vi "UHR-Fleezers Control (host) -Leonardo 04-2018 V2.vi"(0 "Tab Control":T5(tab)=enum."Trap Control (RF)") -> ()   [LabVIEW 2013] (continued)
        n486 = xnode "Read/Write Control"("FPGA VI Reference In"=w836, "error in"=w835, "+ phase"=w832) -> ("error out"=w831:errorcluster)  [unwired: 1 out]
      }
      event "Signals to Plot": Double Click {
        w844 = u32 9868950 ("Color Box")
        n487 = event-data() -> ("Row"=w846:i32)  [unwired: 9 out]
        n488 = property on="All Signals" class="WFChart (strict)"("Active Plot"=w846) -> (error out=w857:errorcluster)  [unwired: 2 in, 1 out]
        n489 = property on="All Signals" class="WFChart (strict)" props=["Plot", "Visible?", "Plot", "Plot Color"](error in=w857) -> (error out=w856:errorcluster, "Plot.Visible?"=w855:bool)  [unwired: 1 in, 2 out]
        n490 = Select(t=FALSE ("Plot.Visible"), s=w855, f=TRUE ("Plot.Visible")) -> (s? t:f=w850:bool)
        n491 = property on="All Signals" class="WFChart (strict)"(error in=w856, "Plot.Visible?"=w850) -> (error out=w852:errorcluster)  [unwired: 1 in, 1 out]
        n492 = property on="All Signals" class="WFChart (strict)"(error in=w852) -> (error out=w847:errorcluster, "Plot.Plot Color"=w851:u32)  [unwired: 1 in, 1 out]
        n493 = property on="Signals to Plot" class="LstBox (strict)"(error in=w847, "Active Row"=w846) -> (error out=w845:errorcluster)  [unwired: 1 in, 1 out]
        n494 = Select(t=w851, s=w850, f=u32 0) -> (s? t:f=w848:u32)
        n495 = property on="Signals to Plot" class="LstBox (strict)"(error in=w845, "CellFontColor"=w848, "SelColor"=w844, "CellBG"=w844, "CellFontSize"=u32 20 ("Active Row:Cell Font:Size"), "CellFontBold"=TRUE ("Active Row:Cell Font:Bold")) -> ()  [unwired: 1 in, 2 out]
      }
      event "Dynamic Force FB": Value Change {
        n496 = event-data() -> ()  [unwired: 7 out]
        n497 = xnode "Read/Write Control"("FPGA VI Reference In"=w859, "Dynamic Force FB (Ronen)"="Dynamic Force FB") -> ()  [unwired: 1 in, 2 out]
      }
      event "BD 1 Frequency 1 (MHz)", "BD 1 Frequency 2 (MHz)", "BD 1 Frequency 3 (MHz)", "BD 2 Frequency 1 (MHz)", "BD 2 Frequency 2 (MHz)", "BD 2 Frequency 3 (MHz)", "Trap Delta (MHz)": Value Change {
        # "anytime one of the frequencies is changed, write it to the RF board UNLESS Set 2 is being oscillated. The oscillation\nscript writes the frequencies to the RF board."
        n498 = event-data() -> ("CtlRef"=w862:refnum<vi>)  [unwired: 6 out]
        n499 = control-ref of="Trap Delta (MHz)"() -> (w861:refnum<vi>)
        n500 = Equal?(x=w861, y=w862) -> (x = y?=w860:bool)
        n501 = case shown="False" "Oscillate Set 2" {
          tunnel: w865 -> [w886 _]
          tunnel: [w885 w898] -> w864
          tunnel: w863 -> [w884 w898]
          tunnel: w860 -> [w871 _]
          frame False {
            n502 = case shown="False" "Symmetric manual \ntrap motion" {
              tunnel: ["T2 for asymmetric\n(MHz)" w897] -> w872
              tunnel: "Trap Delta (MHz)" -> [w891 w896]
              tunnel: [w890 w893] -> w868
              frame False {
                n503 = Subtract(x="T2 for asymmetric\n(MHz)", y=w891) -> (x-y=w890:dbl)
              }
              frame True {
                n504 = Divide(x=w896, y=2) -> (x/y=w894:dbl)
                n505 = Subtract(x="Middle freq for \nsymmetric (MHz)", y=w894) -> (x-y=w893:dbl)
                n506 = Add(x="Middle freq for \nsymmetric (MHz)", y=w894) -> (x+y=w897:dbl)
              }
            }
            n507 = local read "BD 1 Frequency 2 (MHz)"() -> (w873:dbl)
            n508 = local write "BD 1 Frequency 1 (MHz)"(w868) -> ()
            n509 = Select(t=w872, s=w871, f=w873) -> (s? t:f=w870:dbl)
            n510 = local read "Y RF Frequency Limits (MHz)"() -> (w874:T16)
            n511 = local read "X RF Frequency Limits (MHz)"() -> (w875:T16)
            n512 = local read "BD 1 Frequency 3 (MHz)"() -> (w887:dbl)
            n513 = local write "BD 1 Frequency 2 (MHz)"(w870) -> ()
            n514 = local read "BD 2 Frequency 1 (MHz)"() -> (w878:dbl)
            n515 = local read "BD 2 Frequency 2 (MHz)"() -> (w877:dbl)
            n516 = local read "BD 2 Frequency 3 (MHz)"() -> (w888:dbl)
            n517 = call "set RF board frequency - interlace.vi"("Board 2 Frequency Limits"=w874, "Board 1 Frequency Limits"=w875, "error in"=w884, "FPGA VI Reference In"=w886, "Board 2 Frequency 3 (MHz)"=w888, "Board 1 Frequency 3 (MHz)"=w887, "Board 2 Frequency 2 (MHz)"=w877, "Board 2 Frequency 1 (MHz)"=w878, "Board 1 Frequency 2 (MHz)"=w870, "Board 1 Frequency 1  (MHz)"=w868) -> ("error out"=w885:errorcluster)  [unwired: 1 out]
            n518 = Subtract(x=w878, y=w877) -> (x-y=w882:dbl)
            n519 = Subtract(x=w870, y=w868) -> (x-y=w883:dbl)
            n520 = Square(x=w882) -> (x^2=w880:dbl)
            n521 = Square(x=w883) -> (x^2=w881:dbl)
            n522 = Add(x=w881, y=w880) -> (x+y=w879:dbl)
            n523 = Square Root(x=w879) -> (sqrt(x)=w876:dbl)
            n524 = local write "Trap Delta (MHz)"(w876) -> ()
            n525 = property on="Initial delta (MHz)" class="DigNum (strict)"("Val(Sgnl)"=w876) -> ()  [unwired: 2 in, 2 out]
          }
          frame True {
          }
        }
      }
      event "Round T1 X": Value Change {
        n526 = event-data() -> ()  [unwired: 7 out]
        n527 = local read "BD 1 Frequency 1 (MHz)"() -> (w901:dbl)
        n528 = Round To Nearest(number=w901) -> (nearest integer value=w900:dbl)
        n529 = property on="BD 1 Frequency 1 (MHz)" class="DigNum (strict)"("Val(Sgnl)"=w900) -> ()  [unwired: 2 in, 2 out]
      }
      event "Round T2 X": Value Change {
        n530 = event-data() -> ()  [unwired: 7 out]
        n531 = local read "BD 1 Frequency 2 (MHz)"() -> (w903:dbl)
        n532 = Round To Nearest(number=w903) -> (nearest integer value=w902:dbl)
        n533 = property on="BD 1 Frequency 2 (MHz)" class="DigNum (strict)"("Val(Sgnl)"=w902) -> ()  [unwired: 2 in, 2 out]
      }
      event "Stop All": Value Change {
        n534 = event-data() -> ()  [unwired: 7 out]
        n535 = call "hamilton_controller.vi"("action"=T21."DISCONNECT") -> ()  [unwired: 10 in, 1 out]
        n536 = local read "Stop All"() -> (w906:bool)
      }
      event "Delayed Interlace Start": Value Change {
        n537 = event-data() -> ()  [unwired: 7 out]
        n538 = flat-sequence {
          frame #0 {
            n539 = Multiply(x="Delay to Interlace (s)", y=1000.0) -> (x*y=w909:dbl)
            n540 = Wait (ms)(milliseconds to wait=w909) -> ()  [unwired: 1 out]
          }
          frame #1 {
            n541 = property on="Green laser mode" class="RadioBtnsControl (strict)"("Val(Sgnl)"=enum32{"Laser ON", "Laser OFF", "Interlace"}."Interlace" ("Value (Signaling)")) -> ()  [unwired: 2 in, 2 out]
          }
        }
      }
      event "BD 1 Amplitude 1 (%)", "BD 1 Amplitude 2 (%)", "BD 1 Amplitude 3 (%)", "BD 2 Amplitude 1 (%)", "BD 2 Amplitude 2 (%)", "BD 2 Amplitude 3 (%)", "Trap 1 ON", "Trap 2 ON", "Trap 3 ON", "Feedback On/Off", "All FB On/Off": Value Change {
        w933 = i16 1 ("f")
        n542 = event-data() -> ()  [unwired: 7 out]
        n543 = local write "Trap 1 (ON/OFF)"("Trap 1 ON") -> ()
        n544 = local write "Trap 2 (ON/OFF)"("Trap 2 ON") -> ()
        n545 = Boolean To (0,1)(Boolean="Trap 3 ON") -> (0, 1=w934:i16)
        n546 = Boolean To (0,1)(Boolean="Trap 1 ON") -> (0, 1=w935:i16)
        n547 = Boolean To (0,1)(Boolean="Trap 2 ON") -> (0, 1=w936:i16)
        n548 = Select(t=w936, s="Trap ON/OFF X or Y Amp?", f=w933) -> (s? t:f=w931:i16)
        n549 = Select(t=w935, s="Trap ON/OFF X or Y Amp?", f=w933) -> (s? t:f=w932:i16)
        n550 = Select(t=w934, s="Trap ON/OFF X or Y Amp?", f=w933) -> (s? t:f=w930:i16)
        n551 = Select(t=w933, s="Trap ON/OFF X or Y Amp?", f=w936) -> (s? t:f=w928:i16)
        n552 = Select(t=w933, s="Trap ON/OFF X or Y Amp?", f=w935) -> (s? t:f=w929:i16)
        n553 = Select(t=w933, s="Trap ON/OFF X or Y Amp?", f=w934) -> (s? t:f=w927:i16)
        n554 = And(x="All FB On/Off", y="Feedback On/Off") -> (x .and. y?=w925:cluster{"Set 1":bool, "Set 2":bool})
        n555 = local read "BD 1 Amplitude 1 (%)"() -> (w945:dbl)
        n556 = local read "BD 1 Amplitude 2 (%)"() -> (w944:dbl)
        n557 = local read "BD 1 Amplitude 3 (%)"() -> (w943:dbl)
        n558 = Unbundle By Name(w925) -> ("Set 1"=w921:bool, "Set 2"=w918:bool)
        n559 = local read "Y RF Amplitude Limits (%)"() -> (w914:T16)
        n560 = local read "X RF Amplitude Limits (%)"() -> (w915:T16)
        n561 = local read "BD 2 Amplitude 1 (%)"() -> (w946:dbl)
        n562 = local read "BD 2 Amplitude 2 (%)"() -> (w947:dbl)
        n563 = local read "BD 2 Amplitude 3 (%)"() -> (w948:dbl)
        n564 = And(x="Trap 2 ON", y=w918) -> (x .and. y?=w916:bool)
        n565 = And(x="Trap 1 ON", y=w921) -> (x .and. y?=w919:bool)
        n566 = Multiply(x=w932, y=w945) -> (x*y=w940:dbl)
        n567 = Multiply(x=w944, y=w931) -> (x*y=w938:dbl)
        n568 = Multiply(x=w943, y=w930) -> (x*y=w939:dbl)
        n569 = Multiply(x=w946, y=w929) -> (x*y=w949:dbl)
        n570 = Multiply(x=w947, y=w928) -> (x*y=w950:dbl)
        n571 = Multiply(x=w948, y=w927) -> (x*y=w951:dbl)
        n572 = call "set RF board amplitude - interlace.vi"("Board 2 Amplitude Limits"=w914, "Board 1 Amplitude Limits"=w915, "error in"=w941, "FPGA VI Reference In"=w942, "Board 2 Amplitude 3 (%)"=w951, "Board 1 Amplitude 3 (%)"=w939, "Board 2 Amplitude 2 (%)"=w950, "Board 2 Amplitude 1 (%)"=w949, "Board 1 Amplitude 2 (%)"=w938, "Board 1 Amplitude 1 (%)"=w940) -> ("error out"=w923:errorcluster, "FPGA VI Reference Out"=w924:T20)
        n573 = xnode "Read/Write Control"("FPGA VI Reference In"=w924, "error in"=w923, "FB On/Off Set 1"=w919, "FB On/Off Set 2"=w916) -> ("error out"=w922:errorcluster)  [unwired: 1 out]
        n574 = case shown="True" "All FB On/Off" {
          frame False {
          }
          frame True {
            n575 = local write "Feedback overload"(FALSE) -> ()
          }
        }
      }
      event "Load parameters": Value Change {
        n576 = event-data() -> ()  [unwired: 7 out]
        n577 = property on="Saved AOD Raster Scan Parameter Sets" class="Arr (strict)"() -> ("Index Values"=w963:u32[])  [unwired: 2 in, 2 out]
        n578 = Index Array(array=w963, index=0) -> (element=w960:u32)
        n579 = local write "Load parameters"(FALSE ("Load parameters")) -> ()
        n580 = Index Array(array="Saved AOD Raster Scan Parameter Sets", index=w960) -> (element=w959:T31)
        n581 = Unbundle By Name(w959) -> ("Scan Range AOD (nm) 2"=w958:dbl, "Step Size AOD (nm) 2"=w957:dbl, "Scan Speed AOD (nm/s) 2"=w956:dbl, "Number of scans (AOD) 2"=w955:u16)
        n582 = flat-sequence {
          tunnel: w958 -> [w966]
          tunnel: w957 -> [w965]
          tunnel: w956 -> [w964]
          tunnel: w955 -> [w967]
          frame #0 {
            n583 = local write "Scan Speed (nm/s)"(w964) -> ()
            n584 = local write "Scan Range (nm)"(w966) -> ()
            n585 = local write "Step Size (nm)"(w965) -> ()
          }
          frame #1 {
            n586 = property on="Number of F/B Scans (AOD)" class="DigNum (strict)"("Val(Sgnl)"=w967) -> ()  [unwired: 2 in, 2 out]
          }
        }
      }
      event "Trap 1 (ON/OFF)", "Trap 2 (ON/OFF)": Value Change {
        n587 = event-data() -> ()  [unwired: 7 out]
        n588 = property on="Trap 2 ON" class="Bool (strict)"("Val(Sgnl)"="Trap 2 (ON/OFF)") -> ()  [unwired: 2 in, 2 out]
        n589 = property on="Trap 1 ON" class="Bool (strict)"("Val(Sgnl)"="Trap 1 (ON/OFF)") -> ()  [unwired: 2 in, 2 out]
      }
      event "DIO count 1 (ticks)", "DIO count 2 (ticks)", "DIO count 3 (ticks)", "Interlace", "Number Interlace Sets", "Not-Interlacing Set": Value Change {
        n590 = event-data() -> ()  [unwired: 7 out]
        n591 = local read "DIO count 3 (ticks)"() -> (w980:u32)
        n592 = local read "DIO count 1 (ticks)"() -> (w982:u32)
        n593 = local read "DIO count 2 (ticks)"() -> (w981:u32)
        n594 = To Unsigned Byte Integer(number="Not-Interlacing Set") -> (unsigned 8bit integer=w971:u8)
        n595 = Add(x=w971, y=u8 1) -> (x+y=w975:u8)
        n596 = xnode "Read/Write Control"("FPGA VI Reference In"=w986, "error in"=w984, "DIO count 1 (ticks)"=w982, "DIO count 2 (ticks)"=w981, "DIO count 3 (ticks)"=w980, "Interlace ON/OFF"="Interlace", "Number Interlace Cycles"="Number Interlace Sets", "Interlace Off Parameters"=w975) -> ("error out"=w985:errorcluster)  [unwired: 1 out]
        n597 = Build Array(w982, w981, w980) -> (w973:u32[])
        n598 = Split 1D Array(array=w973, index="Number Interlace Sets") -> (first subarray=w983:u32[])  [unwired: 1 out]
        n599 = Index Array(array=w973, index=w971) -> (element=w972:u32)
        n600 = Add Array Elements(numeric array=w983) -> (sum=w977:u32)
        n601 = Select(t=w977, s="Interlace", f=w972) -> (s? t:f=→"Total Counts (ticks)":u32)
      }
      event "Reset Feedback": Value Change {
        n602 = event-data() -> ()  [unwired: 7 out]
        n603 = Unbundle By Name("Reset Feedback") -> ("Set 1"=w990:bool, "Set 2"=w989:bool)
        n604 = xnode "Read/Write Control"("FPGA VI Reference In"=w992, "error in"=w987, "FB Reset Set 1"=w990, "FB Reset Set 2"=w989) -> ("error out"=w988:errorcluster)  [unwired: 1 out]
      }
      event "PID gains": Value Change {
        n605 = event-data() -> ()  [unwired: 7 out]
        n606 = local read "PID gains"() -> (w993:T10)
        n607 = xnode "Read/Write Control"("FPGA VI Reference In"=w996, "error in"=w994, "FB Gains"=w993) -> ("error out"=w995:errorcluster)  [unwired: 1 out]
      }
      event "AI2 to Setpoint", "Trap Intensity\nSetpoints (V)": Value Change {
        n608 = event-data() -> ()  [unwired: 7 out]
        n609 = xnode "Read/Write Control"("FPGA VI Reference In"=w1001, "error in"=w997) -> ("FPGA VI Reference Out"=w1000:T20, "error out"=w999:errorcluster, "AI2 Y Sum Set 1"=w1008:i16, "AI2 Y Sum Set 2"=w1007:i16)
        n610 = Cluster To Array(cluster="AI2 to Setpoint") -> (array=w1011:bool[])
        n611 = local read "AI2 (V)"() -> (w1009:cluster{"Set 1":dbl, "Set 2":dbl})
        n612 = Or Array Elements(Boolean array=w1011) -> (logical OR=w1012:bool)
        n613 = Bundle By Name(cluster=w1009, "Set 1"=w1008, "Set 2"=w1007) -> (w1006:cluster{"Set 1":dbl, "Set 2":dbl})
        n614 = Divide(x=w1006, y=3276.7) -> (x/y=w1005:cluster{"Set 1":dbl, "Set 2":dbl})
        "AI2 (V)" <- w1005
        n615 = case shown="False" w1012 {
          tunnel: [w1015 w1032] -> w1004
          tunnel: "AI2 to Setpoint" -> [_ w1028]
          tunnel: "Trap Intensity\nSetpoints (V)" -> [w1016 w1031]
          tunnel: w1005 -> [_ w1025]
          frame False {
            n616 = Multiply(x=3276.7, y=w1016) -> (x*y=w1017:cluster{"Set 1":dbl, "Set 2":dbl})
            n617 = To Word Integer(number=w1017) -> (16bit integer=w1015:cluster{"Set 1":i16, "Set 2":i16})
          }
          frame True {
            n618 = Unbundle By Name(w1025) -> ("Set 1"=w1024:dbl, "Set 2"=w1023:dbl)
            n619 = Unbundle By Name(w1031) -> ("Set 1"=w1030:dbl, "Set 2"=w1029:dbl)
            n620 = Unbundle By Name(w1028) -> ("Set 1"=w1027:bool, "Set 2"=w1026:bool)
            n621 = Select(t=w1024, s=w1027, f=w1030) -> (s? t:f=w1022:dbl)
            n622 = Select(t=w1023, s=w1026, f=w1029) -> (s? t:f=w1021:dbl)
            n623 = Bundle By Name(cluster=w1031, "Set 1"=w1022, "Set 2"=w1021) -> (w1019:cluster{"Set 1":dbl, "Set 2":dbl})
            n624 = local write "Trap Intensity\nSetpoints (V)"(w1019) -> ()
            n625 = Multiply(x=3276.7, y=w1019) -> (x*y=w1020:cluster{"Set 1":dbl, "Set 2":dbl})
            n626 = To Word Integer(number=w1020) -> (16bit integer=w1032:cluster{"Set 1":i16, "Set 2":i16})
          }
        }
        n627 = Unbundle By Name(w1004) -> ("Set 1"=w1003:i16, "Set 2"=w1002:i16)
        n628 = xnode "Read/Write Control"("FPGA VI Reference In"=w1000, "error in"=w999, "FB Setpoint Set 1"=w1003, "FB Setpoint Set 2"=w1002) -> ("error out"=w998:errorcluster)  [unwired: 1 out]
      }
      event "Invert GI": Value Change {
        n629 = event-data() -> ()  [unwired: 7 out]
        n630 = xnode "Read/Write Control"("FPGA VI Reference In"=w1037, "error in"=w1035, "Invert GI"="Invert GI", "Invert GI 2"="Invert GI") -> ("error out"=w1036:errorcluster)  [unwired: 1 out]
      }
      event "Green FB Setpoint (mV)", "Green FB Gains", "Green FB On/Off", "Current When FB OFF (%)", "Green int current ON count adj": Value Change {
        n631 = event-data() -> ()  [unwired: 7 out]
        n632 = local read "Green FB Setpoint (mV)"() -> (w1044:dbl)
        n633 = local read "Current When FB OFF (%)"() -> (w1047:dbl)
        n634 = Multiply(x=w1044, y=3.2767) -> (x*y=w1043:dbl)
        n635 = Multiply(x=w1047, y=655.35) -> (x*y=w1048:dbl)
        n636 = To Unsigned Word Integer(number=w1048) -> (unsigned 16bit integer=w1046:u16)
        n637 = local read "Green int current ON count adj"() -> (w1051:u32)
        n638 = local read "Green FB Gains"() -> (w1050:T10)
        n639 = local read "Green Laser ON/Interlacing"() -> (w1041:bool)
        n640 = local read "Green laser mode"() -> (w1040:enum32{"Laser ON", "Laser OFF", "Interlace"})
        n641 = local read "Green FB On/Off"() -> (w1052:bool)
        n642 = Equal?(x=w1040, y=enum32{"Laser ON", "Laser OFF", "Interlace"}."Interlace") -> (x = y?=w1038:bool)
        n643 = Compound Arithmetic op=AND(w1038, w1052, w1041) -> (w1042:bool)
        n644 = xnode "Read/Write Control"("FPGA VI Reference In"=w1055, "error in"=w1054, "Green FB Setpoint"=w1043, "Green FB On/Off"=w1042, "Current Out"=w1046, "Green int current ON count adj"=w1051, "Green FB Gains"=w1050) -> ("error out"=w1053:errorcluster)  [unwired: 1 out]
      }
      event "Green laser mode", "Green Laser ON/Interlacing": Value Change {
        n645 = event-data() -> ()  [unwired: 7 out]
        n646 = case shown="True" "Green Laser ON/Interlacing" {
          tunnel: "Green laser mode" -> [_ w1069]
          tunnel: [enum32{"Laser ON", "Laser OFF", "Interlace"}."Laser OFF" ("Green laser mode") w1069] -> w1057
          tunnel: [FALSE w1065] -> w1056
          frame False {
          }
          frame True {
            n647 = local read "Green FB On/Off"() -> (w1066:bool)
            n648 = Equal?(x=w1069, y=enum32{"Laser ON", "Laser OFF", "Interlace"}."Interlace") -> (x = y?=w1067:bool)
            n649 = And(x=w1067, y=w1066) -> (x .and. y?=w1065:bool)
          }
        }
        n650 = xnode "Read/Write Control"("FPGA VI Reference In"=w1062, "error in"=w1060, "Operating Mode"=w1057, "Operating Mode 2"=w1057, "Green FB On/Off"=w1056) -> ("error out"=w1061:errorcluster)  [unwired: 1 out]
      }
      event "- phase (APD 1 Gate)", "+ phase (APD 1 Gate)": Value Change {
        n651 = event-data() -> ()  [unwired: 7 out]
        n652 = local read "Phase Adj. (APD 1 Gate)"() -> (w1070:i16)
        n653 = Negate(x=w1070) -> (-x=w1078:i16)
        n654 = Select(t=w1078, s="- phase (APD 1 Gate)", f=w1070) -> (s? t:f=w1077:i16)
        n655 = Or(x="- phase (APD 1 Gate)", y="+ phase (APD 1 Gate)") -> (x .or. y?=w1073:bool)
        n656 = xnode "Read/Write Control"("FPGA VI Reference In"=w1080, "error in"=w1079, "Phase count adjustment (APD 1 Gate)"=w1077) -> ("FPGA VI Reference Out"=w1075:T20, "error out"=w1076:errorcluster)
        n657 = xnode "Read/Write Control"("FPGA VI Reference In"=w1075, "error in"=w1076, "+ phase (APD 1 Gate)"=w1073) -> ("error out"=w1074:errorcluster)  [unwired: 1 out]
      }
      event "Phase Adj. (APD Acq)", "+ phase (APD Acq)", "- phase (APD Acq)": Value Change {
        n658 = event-data() -> ()  [unwired: 7 out]
        n659 = local read "Phase Adj. (APD Acq)"() -> (w1083:i16)
        n660 = Negate(x=w1083) -> (-x=w1089:i16)
        n661 = Select(t=w1089, s="+ phase (APD Acq)", f=w1083) -> (s? t:f=w1088:i16)
        n662 = Or(x="+ phase (APD Acq)", y="- phase (APD Acq)") -> (x .or. y?=w1084:bool)
        n663 = xnode "Read/Write Control"("FPGA VI Reference In"=w1091, "error in"=w1090, "Phase Count Adjustment (APD Acq)"=w1088) -> ("FPGA VI Reference Out"=w1086:T20, "error out"=w1087:errorcluster)
        n664 = xnode "Read/Write Control"("FPGA VI Reference In"=w1086, "error in"=w1087, "+ phase (APD Acq)"=w1084) -> ("error out"=w1085:errorcluster)  [unwired: 1 out]
      }
      event "Phase adj. (GI)", "+ phase (GI)", "- phase (GI)": Value Change {
        n665 = event-data() -> ()  [unwired: 7 out]
        n666 = Negate(x="Phase adj. (GI)") -> (-x=w1100:i16)
        n667 = Select(t=w1100, s="+ phase (GI)", f="Phase adj. (GI)") -> (s? t:f=w1099:i16)
        n668 = Or(x="+ phase (GI)", y="- phase (GI)") -> (x .or. y?=w1095:bool)
        n669 = xnode "Read/Write Control"("FPGA VI Reference In"=w1102, "error in"=w1101, "Phase count adjustment (GI)"=w1099) -> ("FPGA VI Reference Out"=w1097:T20, "error out"=w1098:errorcluster)
        n670 = xnode "Read/Write Control"("FPGA VI Reference In"=w1097, "error in"=w1098, "+ phase (GI)"=w1095) -> ("error out"=w1096:errorcluster)  [unwired: 1 out]
      }
      event "Phase adj. (GI) 2", "+ phase (GI) 2", "- phase (GI) 2": Value Change {
        n671 = event-data() -> ()  [unwired: 7 out]
        n672 = Negate(x="Phase adj. (GI) 2") -> (-x=w1111:i16)
        n673 = Select(t=w1111, s="+ phase (GI) 2", f="Phase adj. (GI) 2") -> (s? t:f=w1110:i16)
        n674 = Or(x="+ phase (GI) 2", y="- phase (GI) 2") -> (x .or. y?=w1106:bool)
        n675 = xnode "Read/Write Control"("FPGA VI Reference In"=w1113, "error in"=w1112, "Phase count adjustment (GI) 2"=w1110) -> ("FPGA VI Reference Out"=w1108:T20, "error out"=w1109:errorcluster)
        n676 = xnode "Read/Write Control"("FPGA VI Reference In"=w1108, "error in"=w1109, "+ phase (GI) 2"=w1106) -> ("error out"=w1107:errorcluster)  [unwired: 1 out]
      }
      event "Phase adj. (Green FB)", "- phase (Green FB)", "+ phase (Green FB)": Value Change {
        n677 = event-data() -> ()  [unwired: 7 out]
        n678 = Negate(x="Phase adj. (Green FB)") -> (-x=w1122:i16)
        n679 = Select(t=w1122, s="+ phase (Green FB)", f="Phase adj. (Green FB)") -> (s? t:f=w1121:i16)
        n680 = Or(x="+ phase (Green FB)", y="- phase (Green FB)") -> (x .or. y?=w1117:bool)
        n681 = xnode "Read/Write Control"("FPGA VI Reference In"=w1124, "error in"=w1123, "Phase count adjustment (Green FB)"=w1121) -> ("FPGA VI Reference Out"=w1119:T20, "error out"=w1120:errorcluster)
        n682 = xnode "Read/Write Control"("FPGA VI Reference In"=w1119, "error in"=w1120, "+ phase (Green FB)"=w1117) -> ("error out"=w1118:errorcluster)  [unwired: 1 out]
      }
      event "Invert APD Gate", "APD Gate ON Count", "APD Gate OFF Count", "APD Gate", "APD Integration Time (s)", "APD 1 AO Mult.", "APD 2 AO Mult.": Value Change {
        n683 = event-data() -> ()  [unwired: 7 out]
        n684 = local read "APD Integration Time (s)"() -> (w1125:dbl)
        n685 = local read "APD Gate ON Count"() -> (w1138:u32)
        n686 = local read "APD Gate OFF Count"() -> (w1137:u32)
        n687 = local read "Invert APD Gate"() -> (w1139:bool)
        n688 = local read "APD Gate"() -> (w1136:enum32{"ON", "OFF", "Interlace"})
        n689 = Multiply(x=w1125, y=40000000.0) -> (x*y=w1134:dbl)
        n690 = Reciprocal(x=w1125) -> (1/x=→"APD Acq Rate (Hz)":dbl)
        n691 = To Unsigned Long Integer(number=w1134) -> (unsigned 32bit integer=w1133:u32)
        n692 = local read "DMA Update Period (s)"() -> (w1126:dbl)
        n693 = Divide(x=w1126, y=w1125) -> (x/y=w1129:dbl)
        n694 = local read "APD 1 AO Mult."() -> (w1131:i16)
        n695 = local read "APD 2 AO Mult."() -> (w1130:i16)
        n696 = Multiply(x=2.0, y=w1129) -> (x*y=w1128:dbl)
        n697 = local write "APD Samples/FIFO Acq."(w1129) -> ()
        n698 = local write "APD Elements/DMA read"(w1128) -> ()
        n699 = xnode "Read/Write Control"("FPGA VI Reference In"=w1142, "error in"=w1141, "Invert APD Gate"=w1139, "APD Gate ON Count"=w1138, "APD Gate OFF Count"=w1137, "APD Acq Rate Count"=w1133, "APD Gate Operating Mode"=w1136, "APD 1 AO scale factor"=w1131, "APD 2 AO scale factor"=w1130) -> ("error out"=w1140:errorcluster)  [unwired: 1 out]
      }
      event "GI Frequency, ON count", "Green FB Count", "GI Frequency, OFF count": Value Change {
        n700 = event-data() -> ()  [unwired: 7 out]
        n701 = xnode "Read/Write Control"("FPGA VI Reference In"=w1148, "error in"=w1146, "Green interlace ON count"="GI Frequency, ON count", "Green interlace OFF count"="GI Frequency, OFF count", "Green interlace ON count 2"="GI Frequency, ON count", "Green interlace OFF count 2"="GI Frequency, OFF count", "Green FB Count"="Green FB Count") -> ("error out"=w1147:errorcluster)  [unwired: 1 out]
      }
      event "Number of F/B Scans (AOD)", "Scan Speed (nm/s)", "Scan BD", "Initial delta (MHz)", "Step Size (nm)", "Scan Range (nm)": Value Change {
        w1210 = 123.0  # AOM cal (nm/MHz)
        n702 = event-data() -> ()  [unwired: 7 out]
        n703 = local read "BD 1 Frequency 1 (MHz)"() -> (w1193:dbl)
        n704 = local read "AOM X Cal (nm/MHz)"() -> (w1185:dbl)
        n705 = local read "X RF Frequency Limits (MHz)"() -> (w1197:T16)
        n706 = local read "Y RF Frequency Limits (MHz)"() -> (w1194:T16)
        n707 = local read "BD 2 Frequency 1 (MHz)"() -> (w1199:dbl)
        n708 = Negate(x="Scan Range (nm)") -> (-x=w1163:dbl)
        n709 = Divide(x=w1163, y=w1185) -> (x/y=w1167:dbl)
        n710 = Select(t=w1197, s="Scan BD", f=w1194) -> (s? t:f=w1196:T16)
        n711 = Select(t=w1193, s="Scan BD", f=w1199) -> (s? t:f=w1198:dbl)
        n712 = Unbundle By Name(w1196) -> ("Maximum"=w1205:dbl, "Minimum"=w1204:dbl)
        n713 = Add(x=w1167, y=w1198) -> (x+y=w1202:dbl)
        n714 = Divide(x=w1163, y="Step Size (nm)") -> (x/y=w1182:dbl)
        n715 = Divide(x="Step Size (nm)", y=w1185) -> (x/y=w1191:dbl)
        n716 = Absolute Value(x=w1182) -> (abs(x)=w1166:dbl)
        n717 = Sign(1:w1163) -> (0:w1164:dbl)
        n718 = In Range and Coerce(upper limit=w1205, x=w1202, lower limit=w1204) -> (coerced(x)=w1201:dbl, In Range?=w1203:bool)
        n719 = To Unsigned Quad Integer(1:w1166) -> (0:w1181:u64)
        "Scan steps (AOD)" <- w1181
        n720 = call "IR AOM freq to word.vi"("Frequency In (MHz)"=w1191) -> ("Frequency Word Out (double)"=w1188:dbl)
        n721 = Multiply(x=w1164, y=w1188) -> (x*y=w1165:dbl)
        n722 = Subtract(x=w1202, y=w1201) -> (x-y=w1200:dbl)
        n723 = To Quad Integer(1:w1165) -> (0:w1187:i64)
        "Incr. int (AOD)" <- w1187
        n724 = Subtract(x=w1167, y=w1200) -> (x-y=w1186:dbl)
        "Scan Range (MHz)" <- w1186
        n725 = Select(t=w1167, s=w1203, f=w1186) -> (s? t:f=w1206:dbl)
        n726 = Multiply(x=w1186, y=w1185) -> (x*y=w1184:dbl)
        n727 = Decrement(x=w1181) -> (x-1=w1234:u64)
        n728 = Negate(x=w1184) -> (-x=w1180:dbl)
        n729 = local write "Scan Range (nm)"(w1180) -> ()
        n730 = Divide(x=w1206, y=w1234) -> (x/y=w1190:dbl)
        "Scan Increment (MHz)" <- w1190
        n731 = call "IR AOM freq to word.vi"("Frequency In (MHz)"=w1190) -> ("Frequency Word Out (double)"=w1189:dbl)
        n732 = Divide(x="Step Size (nm)", y="Scan Speed (nm/s)") -> (x/y=w1177:dbl)
        n733 = To Quad Integer(1:w1189) -> ()  [unwired: 1 out]
        n734 = local read "Number Interlace Sets"() -> (w1161:u8)
        n735 = local read "AI Count (ticks)"() -> (w1162:u32)
        n736 = local read "Total Counts (ticks)"() -> (w1160:u32)
        n737 = local read "# Samples/trap"() -> (w1192:u32)
        n738 = Multiply(x=w1162, y=w1161) -> (x*y=w1159:u32)
        n739 = Divide(x=w1160, y=w1159) -> (x/y=w1158:dbl)
        n740 = Select(t=w1193, s="Scan BD", f=w1199) -> (s? t:f=w1231:dbl)
        "Initial freq. (MHz)" <- w1231
        n741 = Add(x=w1206, y=w1231) -> (x+y=→"Final freq. (MHz)":dbl)
        n742 = Divide(x=w1160, y=40000000.0) -> (x/y=w1176:dbl)
        n743 = Divide(x=w1177, y=w1176) -> (x/y=w1175:dbl)
        n744 = To Unsigned Quad Integer(1:w1175) -> (0:w1150:u64)
        n745 = Quotient & Remainder(x=w1150, y=u64 2) -> (x-y*floor(x/y)=w1154:u64)  [unwired: 1 out]
        n746 = Equal?(x=w1154, y=u64 0) -> (x = y?=w1152:bool)
        n747 = Decrement(x=w1150) -> (x-1=w1151:u64)
        n748 = Select(t=w1150, s=w1152, f=w1151) -> (s? t:f=w1149:u64)
        "Cycles/step (AOD)" <- w1149
        n749 = xnode "Read/Write Control"("FPGA VI Reference In"=w1242, "error in"=w1241, "Scan steps"=w1181, "Number of scans"="Number of F/B Scans (AOD)", "Cycles per step"=w1149, "Scan freq.  increment"=w1187, "Scan BD"="Scan BD") -> ("error out"=w1240:errorcluster)  [unwired: 1 out]
        n750 = Multiply(x=w1181, y=w1149) -> (x*y=w1235:u64)
        n751 = Multiply(x=w1235, y=u64 2) -> (x*y=w1157:u64)
        n752 = Multiply(x=w1158, y=w1157) -> (x*y=w1156:dbl)
        "Data points/scan (f/b)" <- w1156
        n753 = Multiply(x=w1156, y="Number of F/B Scans (AOD)") -> (x*y=w1238:dbl)
        "Data points/scans" <- w1238
        n754 = Divide(x=w1238, y=w1192) -> (x/y=→"N sets should be saved":dbl)
        n755 = Multiply(x=w1235, y=w1176) -> (x*y=w1174:dbl)
        "Time/Scan (s) (AOD)" <- w1174
        n756 = Select(t=w1206, s="Scan BD", f=0.0) -> (s? t:f=w1232:dbl)
        n757 = Select(t=0.0, s="Scan BD", f=w1206) -> (s? t:f=w1228:dbl)
        n758 = local read "BD 2 Frequency 2 (MHz)"() -> (w1224:dbl)
        n759 = local read "BD 1 Frequency 2 (MHz)"() -> (w1227:dbl)
        n760 = Add(x=w1228, y=w1199) -> (x+y=w1225:dbl)
        n761 = Add(x=w1193, y=w1232) -> (x+y=w1226:dbl)
        n762 = Multiply(x=w1174, y=2.0) -> (x*y=w1173:dbl)
        n763 = Multiply(x=w1173, y="Number of F/B Scans (AOD)") -> (x*y=w1170:dbl)
        n764 = Divide(x=w1170, y=60.0) -> (x/y=→"Time to Finish All (min)":dbl)
        n765 = Add(x="Trap 2 Bead Size (nm)", y="Trap 1 Bead Size (nm)") -> (x+y=w1214:dbl)
        n766 = local read "Initial delta (MHz)"() -> (w1211:dbl)
        n767 = Divide(x=w1214, y=2.0) -> (x/y=w1208:dbl)
        n768 = Subtract(x=w1225, y=w1224) -> (x-y=w1222:dbl)
        n769 = Subtract(x=w1226, y=w1227) -> (x-y=w1223:dbl)
        n770 = Square(x=w1222) -> (x^2=w1221:dbl)
        n771 = Square(x=w1223) -> (x^2=w1220:dbl)
        n772 = Add(x=w1220, y=w1221) -> (x+y=w1219:dbl)
        n773 = Square Root(x=w1219) -> (sqrt(x)=w1218:dbl)
        "Final delta (MHz)" <- w1218
        n774 = Multiply(x=w1210, y=w1218) -> (x*y=w1217:dbl)
        n775 = Multiply(x=w1211, y=w1210) -> (x*y=w1209:dbl)
        n776 = Subtract(x=w1209, y=w1208) -> (x-y=→"Initial sep (nm)":dbl)
        n777 = Subtract(x=w1217, y=w1208) -> (x-y=→"Final sep (nm)":dbl)
      }
      event "Raster Scanning...": Value Change {
        n778 = event-data() -> ("NewVal"=w1243:bool)  [unwired: 6 out]
        n779 = case shown="True" w1243 {
          frame False {
          }
          frame True {
            n780 = property on="BD 1 Frequency 1 (MHz)" class="DigNum (strict)"("Val(Sgnl)"=65.0 ("Value (Signaling)")) -> ()  [unwired: 2 in, 2 out]
          }
        }
      }
      event "Phase increment trap 1", "Swap F1 and F2", "Freq switch delay", "Amp switch delay", "Phase increment trap 2", "RF phase reset before cycles", "Phase offset method": Value Change {
        n781 = event-data() -> ()  [unwired: 7 out]
        n782 = local read "Amp switch delay"() -> (w1249:u16)
        n783 = local read "Phase increment trap 1"() -> (w1248:fxp<+/-,64,32>)
        n784 = local read "Freq switch delay"() -> (w1251:u16)
        n785 = local read "Phase increment trap 2"() -> (w1247:fxp<+/-,64,32>)
        n786 = local read "RF phase reset before cycles"() -> (w1246:bool)
        n787 = local read "Swap F1 and F2"() -> (w1250:bool)
        n788 = local read "Phase offset method"() -> (w1245:u8)
        n789 = xnode "Read/Write Control"("FPGA VI Reference In"=w1254, "error in"=w1253, "BD 1 Delay (ticks)"=w1251, "Swap F1 and F2"=w1250, "Amp switch delay"=w1249, "Phase Trap 1"=w1248, "Phase Trap 2"=w1247, "RF phase reset before cycles"=w1246, "Phase offset method"=w1245) -> ("error out"=w1252:errorcluster)  [unwired: 1 out]
      }
      event "Scan steps (MCL)", "Number of scans (MCL)", "Scan Range (V)\n(of steps)", "2D or 1D Scan", "N APD Samp/step", "Fast Scan Dir", "Continuous MCL Scanning", "Scan lines (y)": Value Change {
        w1256 = 32767.0 ("y")
        n790 = event-data() -> ()  [unwired: 7 out]
        n791 = Select(t="Scan lines (y)", s="2D or 1D Scan", f="Number of scans (MCL)") -> (s? t:f=w1261:u64)
        n792 = Decrement(x="Scan steps (MCL)") -> (x-1=w1277:u64)
        n793 = Divide(x="Scan Range (V)\n(of steps)", y=w1277) -> (x/y=w1276:dbl)
        "Desired Scan Incr (V)" <- w1276
        n794 = local read "APD Integration Time (s)"() -> (w1269:dbl)
        n795 = Multiply(x=w1276, y=w1256) -> (x*y=w1285:dbl)
        n796 = Divide(x=w1285, y=10.0) -> (x/y=w1275:dbl)
        "Desired incr (int)" <- w1275
        n797 = local read "Update Count (MCL)"() -> (w1281:u32)
        n798 = Round Toward -Infinity(1:w1275) -> (0:w1284:dbl)
        n799 = To Word Integer(number=w1284) -> (16bit integer=w1259:i16)
        "Actual Incr. int (MCL)" <- w1259
        n800 = Multiply(x=w1269, y=40000000.0) -> (x*y=w1282:dbl)
        n801 = Divide(x=w1282, y=w1281) -> (x/y=w1280:dbl)
        n802 = Multiply(x=i16 10, y=w1259) -> (x*y=w1257:i16)
        n803 = Multiply(x="N APD Samp/step", y=w1280) -> (x*y=w1279:dbl)
        "Cycles/step (MCL)" <- w1279
        n804 = Divide(x=w1257, y=w1256) -> (x/y=→"Actual MCL Inc (V)":dbl)
        n805 = Multiply(x="N APD Samp/step", y="Scan steps (MCL)") -> (x*y=w1271:dbl)
        n806 = local read "APD Samples/FIFO Acq."() -> (w1268:dbl)
        n807 = Multiply(x=w1271, y=u64 2) -> (x*y=w1270:dbl)
        "Data points/scan (f+b)" <- w1270
        n808 = Multiply(x=w1270, y=w1261) -> (x*y=w1288:dbl)
        "Data points/scans (MCL)" <- w1288
        n809 = Multiply(x=w1269, y=w1270) -> (x*y=w1262:dbl)
        "Time/f+b scan (s) (MCL)" <- w1262
        n810 = Divide(x=w1288, y=w1268) -> (x/y=→"N sets should be saved (MCL)":dbl)
        n811 = Multiply(x=w1262, y=w1261) -> (x*y=→"Total Time (s)":dbl)
        n812 = Not(x="Fast Scan Dir") -> (.not. x?=w1266:bool)
        n813 = xnode "Read/Write Control"("FPGA VI Reference In"=w1292, "error in"=w1291, "Scan steps (MCL)"="Scan steps (MCL)", "Number of scans (MCL)"=w1261, "Cycles per step (MCL)"=w1279, "Scan freq.  increment (MCL)"=w1259, "1D or 2D Scan?"="2D or 1D Scan", "MCL Scan Axis"=w1266, "Cont. Scan (MCL)"="Continuous MCL Scanning") -> ("error out"=w1290:errorcluster)  [unwired: 1 out]
      }
      event "Read Cal": Value Change {
        w1325 = 1000.0 ("y")
        w1313 = T30."big-endian, network order" ("byte order (0:big-endian, network order)")
        w1314 = -1 ("count (1)")
        n814 = event-data() -> ()  [unwired: 7 out]
        n815 = local read "Save file name"() -> (w1343:path)
        n816 = local write "Read Cal"(FALSE ("Read Cal")) -> ()
        n817 = Strip Path(path=w1343) -> (stripped path=w1342:path)  [unwired: 1 out]
        n818 = Path To String(path=w1342) -> (string=w1323:string)
        n819 = Concatenate Strings(w1323, "\\current.off" ("string")) -> (w1321:string)
        n820 = Concatenate Strings(w1323, "\\current.cal" ("string")) -> (w1340:string)
        n821 = String To Path(string=w1340) -> (path=w1339:path)
        n822 = String To Path(string=w1321) -> (path=w1320:path)
        n823 = Open/Create/Replace File(file path (use dialog)=w1339, operation (0:open)=T24."open", access (0:read/write)=enum16{"read/write", "read-only", "write-only"}."read-only") -> (refnum out=w1346:refnum<file>, error out=w1335:errorcluster)  [unwired: 1 in, 3 out]
        n824 = Deny Access(4:w1335, 7:w1346) -> (0:w1334:errorcluster, 3:w1338:refnum<file>)  [unwired: 1 out]
        n825 = Open/Create/Replace File(file path (use dialog)=w1320, operation (0:open)=T24."open", access (0:read/write)=enum16{"read/write", "read-only", "write-only"}."read-only") -> (refnum out=w1317:refnum<file>)  [unwired: 1 in, 4 out]
        n826 = Deny Access(7:w1317) -> (3:w1315:refnum<file>)  [unwired: 1 in, 2 out]
        n827 = Read from Binary File(5:0.0, 8:w1334, 9:w1313, 10:w1314, 11:w1338) -> (0:w1333:errorcluster, 2:w1331:dbl[], 3:w1336:refnum<file>)  [unwired: 2 out]
        n828 = Array To Cluster(array=w1331) -> (cluster=w1330:T32)
        n829 = Unbundle(w1330) -> ("[0]"=w1304:dbl, "[1]"=w1302:dbl, "[2]"=w1303:dbl, "[3]"=w1301:dbl, "[4]"=w1329:dbl, "[5]"=w1328:dbl)
        n830 = Close File(refnum=w1336, error in=w1333) -> (error out=→"Read cal error":errorcluster)  [unwired: 1 out]
        n831 = Multiply(x=w1328, y=w1325) -> (x*y=w1326:dbl)
        n832 = local write "T2 kappa_x (pN/nm)"(w1301) -> ()
        n833 = local write "T1 kappa_x (pN/nm)"(w1303) -> ()
        n834 = local write "T1 alpha_x (nm/V)"(w1304) -> ()
        n835 = local write "T2 alpha_x (nm/V)"(w1302) -> ()
        n836 = Read from Binary File(5:0.0, 9:w1313, 10:w1314, 11:w1315) -> (2:w1309:dbl[], 3:w1312:refnum<file>)  [unwired: 1 in, 3 out]
        n837 = Multiply(x=w1329, y=w1325) -> (x*y=w1327:dbl)
        n838 = local write "T1 offset_x (mV)"(w1327) -> ()
        n839 = local write "T2 offset_x (mV)"(w1326) -> ()
        n840 = Close File(refnum=w1312) -> ()  [unwired: 1 in, 2 out]
        n841 = Array Subset(array=w1309, index=3) -> (w1307:dbl[])  [unwired: 1 in]
        n842 = Index Array(array=w1309, index=0) -> (element=→"Offset file step size":dbl)
        n843 = Multiply(x=w1304, y=w1303) -> (x*y=w1299:dbl)
        n844 = Multiply(x=w1302, y=w1301) -> (x*y=w1300:dbl)
        n845 = Divide(x=w1300, y=w1299) -> (x/y=w1294:dbl)
        n846 = Decimate 1D Array(w1307) -> (w1297:dbl[], w1298:dbl[])  [unwired: 1 out]
        n847 = property on="B factor" class="DigNum (strict)"("Val(Sgnl)"=w1294) -> ()  [unwired: 2 in, 2 out]
        n848 = Bundle By Name(cluster="Offset Values", "Trap 1X offset"=w1297, "Trap 2X offset"=w1298) -> (w1305:T14)
        n849 = Multiply(x=w1298, y=w1294) -> (x*y=w1296:dbl[])
        n850 = Subtract(x=w1297, y=w1296) -> (x-y=w1295:dbl[])
        n851 = local write "Offset Values"(w1305) -> ()
        n852 = case shown="True" "Auto read offset\ncorrection" {
          tunnel: w1295 -> [_ w1347]
          frame False {
          }
          frame True {
            n853 = property on="Setpoint offset\nCorrection values" class="Arr (strict)"("Val(Sgnl)"=w1347) -> ()  [unwired: 2 in, 2 out]
          }
        }
      }
      event "Abort MCL Scan": Value Change {
        n854 = event-data() -> ()  [unwired: 7 out]
        n855 = local write "MCL Scanning"(FALSE ("MCL Scanning")) -> ()
        n856 = xnode "Read/Write Control"("FPGA VI Reference In"=w1352, "error in"=w1351, "Abort scan (MCL)"="Abort MCL Scan") -> ("error out"=w1350:errorcluster)  [unwired: 1 out]
      }
      event "Update Count (MCL)": Value Change {
        n857 = event-data() -> ()  [unwired: 7 out]
        n858 = xnode "Read/Write Control"("FPGA VI Reference In"=w1356, "error in"=w1355, "MCL count"="Update Count (MCL)") -> ("error out"=w1354:errorcluster)  [unwired: 1 out]
      }
      event "Phase adjust (MCL)", "+ phase (MCL)", "- phase (MCL)": Value Change {
        n859 = event-data() -> ()  [unwired: 7 out]
        n860 = Negate(x="Phase adjust (MCL)") -> (-x=w1365:i16)
        n861 = Select(t=w1365, s="- phase (MCL)", f="Phase adjust (MCL)") -> (s? t:f=w1363:i16)
        n862 = Or(x="- phase (MCL)", y="+ phase (MCL)") -> (x .or. y?=w1358:bool)
        n863 = xnode "Read/Write Control"("FPGA VI Reference In"=w1367, "error in"=w1366, "Phase count adjustment (MCL)"=w1363) -> ("FPGA VI Reference Out"=w1359:T20, "error out"=w1360:errorcluster)
        n864 = xnode "Read/Write Control"("FPGA VI Reference In"=w1359, "error in"=w1360, "+ phase (MCL)"=w1358) -> ("error out"=w1357:errorcluster)  [unwired: 1 out]
      }
      event "Abort AOD Scan": Value Change {
        n865 = event-data() -> ()  [unwired: 7 out]
        n866 = flat-sequence {
          tunnel: w1372 -> [w1379]
          tunnel: w1371 -> [w1378]
          tunnel: [w1377] -> w1369
          tunnel: [w1373] -> w1368
          tunnel: [w1392] -> w1370
          tunnel: w1369 -> [w1392]
          tunnel: w1368 -> [w1391]
          frame #0 {
            n867 = local read "Save scans"() -> (w1375:bool)
            n868 = xnode "Read/Write Control"("FPGA VI Reference In"=w1379, "error in"=w1378, "Abort scan"="Abort AOD Scan") -> ("FPGA VI Reference Out"=w1373:T20, "error out"=w1377:errorcluster)
            n869 = local write "Raster Scanning..."(FALSE) -> ()
            n870 = case shown="True" w1375 {
              frame False {
              }
              frame True {
                n871 = local write "Stop Saving"(TRUE) -> ()
              }
            }
          }
          frame #1 {
            n872 = xnode "Read/Write Control"("FPGA VI Reference In"=w1391) -> ("BD1 Frequency Out 1"=w1382:u64)  [unwired: 1 in, 2 out]
            n873 = To Double Precision Float(number=w1382) -> (double precision float=w1388:dbl)
            n874 = Multiply(x=49125000.0, y=6.0) -> (x*y=w1387:dbl)
            n875 = Multiply(x=w1388, y=w1387) -> (x*y=w1385:dbl)
            n876 = Scale By Power Of 2(n=-48, x=w1385) -> (x*2^n=w1384:dbl)
            n877 = Divide(x=w1384, y=1000000.0) -> (x/y=w1381:dbl)
            n878 = property on="BD 1 Frequency 1 (MHz)" class="DigNum (strict)"("Val(Sgnl)"=w1381) -> ()  [unwired: 2 in, 2 out]
          }
        }
      }
      event "Continuous AOD Scanning": Value Change {
        n879 = event-data() -> ()  [unwired: 7 out]
        n880 = xnode "Read/Write Control"("FPGA VI Reference In"=w1396, "error in"=w1395, "Cont. Scan"="Continuous AOD Scanning") -> ("error out"=w1394:errorcluster)  [unwired: 1 out]
      }
      event "Index": Value Change {
        n881 = event-data() -> ()  [unwired: 7 out]
        n882 = call "Create new save file.vi"("Insert"="", "Ext"=".dat" ("string"), "Index In"="Index") -> ("Path Out"=→"Save file name":path, "Index Out"=w1397:dbl)
        "Save index" <- w1397
        n883 = local write "Index"(w1397) -> ()
      }
      event "AO1", "AO2": Value Change {
        w1412 = 10.0 ("y")
        w1411 = 32767.0 ("y")
        n884 = event-data() -> ()  [unwired: 7 out]
        n885 = local read "AO2"() -> (w1410:dbl)
        n886 = local read "AO1"() -> (w1407:dbl)
        n887 = Multiply(x=w1407, y=w1411) -> (x*y=w1406:dbl)
        n888 = Multiply(x=w1410, y=w1411) -> (x*y=w1409:dbl)
        n889 = Divide(x=w1406, y=w1412) -> (x/y=w1405:dbl)
        n890 = Divide(x=w1409, y=w1412) -> (x/y=w1408:dbl)
        n891 = To Word Integer(number=w1405) -> (16bit integer=w1413:i16)
        n892 = To Word Integer(number=w1408) -> (16bit integer=w1414:i16)
        n893 = xnode "Read/Write Control"("FPGA VI Reference In"=w1404, "error in"=w1403, "AO1 (Y)"=w1413, "AO2 (X)"=w1414) -> ("error out"=w1402:errorcluster)  [unwired: 1 out]
      }
      event "Inject Top:": Value Change {
        n894 = event-data() -> ()  [unwired: 7 out]
        n895 = disable-structure shown="Enabled" {
          disable-tunnel: "Inject Top:" -> [w1416 w1456]
          frame Disabled {
            n896 = local read "Chemyx Syringe Pump Serial Port"() -> (w1417:refnum<visa-resource-name>)
            n897 = local read "Pump write delay (ms)"() -> (w1418:dbl)
            n898 = case shown="True" w1416 {
              tunnel: w1418 -> [w1424 w1438]
              tunnel: w1417 -> [w1421 w1437]
              frame False {
                n899 = flat-sequence {
                  tunnel: w1421 -> [w1425]
                  tunnel: [w1425] -> w1422
                  tunnel: w1424 -> [_]
                  tunnel: [w1428] -> w1423
                  tunnel: w1422 -> [w1428]
                  tunnel: w1423 -> [w1429]
                  tunnel: [w1429] -> w1419
                  tunnel: [w1431] -> w1420
                  tunnel: w1419 -> [w1431]
                  tunnel: w1420 -> [w1433]
                  frame #0 {
                    n900 = call "Write to pump.vi"("string"="enter pump1", "VISA resource name"=w1425) -> ()  [unwired: 1 out]
                  }
                  frame #1 {
                    n901 = Wait (ms)(milliseconds to wait="Pump pause delay (ms)") -> ()  [unwired: 1 out]
                  }
                  frame #2 {
                    n902 = call "Write to pump.vi"("string"="stop", "VISA resource name"=w1429) -> ()  [unwired: 1 out]
                  }
                  frame #3 {
                    n903 = Wait (ms)(milliseconds to wait=u32 500) -> ()  [unwired: 1 out]
                  }
                  frame #4 {
                    n904 = call "Write to pump.vi"("string"="stop", "VISA resource name"=w1433) -> ()  [unwired: 1 out]
                  }
                }
              }
              frame True {
                n905 = flat-sequence {
                  tunnel: w1437 -> [w1447]
                  tunnel: w1438 -> [w1442]
                  tunnel: w1438 -> [w1449]
                  tunnel: w1437 -> [w1450]
                  tunnel: [w1450] -> w1435
                  tunnel: [w1452] -> w1436
                  tunnel: w1435 -> [w1452]
                  tunnel: w1436 -> [w1454]
                  frame #0 {
                    n906 = local read "All Pump Parameters"() -> (w1441:T6)
                    n907 = Unbundle By Name(w1441) -> ("Pump 1"=w1448:T33)
                    n908 = call "Set pump parameters.vi"("Pump write delay (ms)"=w1442, "Volume (uL)"="Ch 2 Inject Volume (uL)", "Rate (uL/h)"="Ch 1 Inject Rate (ul/h)", "Units"=4.0, "Pump #"=1.0, "Pump Parameters In"=w1448, "VISA resource name"=w1447) -> ("Pump Parameters Out"=w1440:T33)  [unwired: 3 in]
                    n909 = Bundle By Name(cluster=w1441, "Pump 1"=w1440) -> (w1439:T6)
                    n910 = local write "All Pump Parameters"(w1439) -> ()
                  }
                  frame #1 {
                    n911 = Wait (ms)(milliseconds to wait=w1449) -> ()  [unwired: 1 out]
                  }
                  frame #2 {
                    n912 = call "Write to pump.vi"("string"="start", "VISA resource name"=w1450) -> ()  [unwired: 1 out]
                  }
                  frame #3 {
                    n913 = Wait (ms)(milliseconds to wait=u32 500) -> ()  [unwired: 1 out]
                  }
                  frame #4 {
                    n914 = call "Write to pump.vi"("string"="start", "VISA resource name"=w1454) -> ()  [unwired: 1 out]
                  }
                }
              }
            }
          }
          frame Enabled {
            n915 = call "hamilton_controller.vi"("Open?"=w1456, "valve"=enum16{"A", "B", "C", "D", "ALL"}."B", "action"=T21."MOVE VALVE") -> ()  [unwired: 8 in, 1 out]
          }
        }
      }
      event "Main:": Value Change {
        n916 = event-data() -> ()  [unwired: 7 out]
        n917 = disable-structure shown="Disabled" {
          disable-tunnel: "Main:" -> [_ w1500]
          frame Disabled {
            n918 = local read "Pump write delay (ms)"() -> (w1461:dbl)
            n919 = case shown="False" w1462 {
              tunnel: w1461 -> [w1468 w1482]
              tunnel: "Chemyx Syringe Pump Serial Port" -> [w1465 w1481]
              frame False {
                n920 = flat-sequence {
                  tunnel: w1465 -> [w1469]
                  tunnel: [w1469] -> w1466
                  tunnel: w1468 -> [_]
                  tunnel: [w1472] -> w1467
                  tunnel: w1466 -> [w1472]
                  tunnel: w1467 -> [w1473]
                  tunnel: [w1473] -> w1463
                  tunnel: [w1475] -> w1464
                  tunnel: w1463 -> [w1475]
                  tunnel: w1464 -> [w1477]
                  frame #0 {
                    n921 = call "Write to pump.vi"("string"="enter pump3", "VISA resource name"=w1469) -> ()  [unwired: 1 out]
                  }
                  frame #1 {
                    n922 = local read "Pump pause delay (ms)"() -> (w1471:u32)
                    n923 = Wait (ms)(milliseconds to wait=w1471) -> ()  [unwired: 1 out]
                  }
                  frame #2 {
                    n924 = call "Write to pump.vi"("string"="stop", "VISA resource name"=w1473) -> ()  [unwired: 1 out]
                  }
                  frame #3 {
                    n925 = Wait (ms)(milliseconds to wait=u32 0) -> ()  [unwired: 1 out]
                  }
                  frame #4 {
                    n926 = call "Write to pump.vi"("string"="stop", "VISA resource name"=w1477) -> ()  [unwired: 1 out]
                  }
                }
              }
              frame True {
                n927 = flat-sequence {
                  tunnel: w1481 -> [w1491]
                  tunnel: w1482 -> [w1486]
                  tunnel: w1482 -> [w1493]
                  tunnel: w1481 -> [w1494]
                  tunnel: [w1494] -> w1479
                  tunnel: [w1497] -> w1480
                  tunnel: w1479 -> [w1497]
                  tunnel: w1480 -> [w1498]
                  frame #0 {
                    n928 = local read "All Pump Parameters"() -> (w1485:T6)
                    n929 = Unbundle By Name(w1485) -> ("Pump 3"=w1492:T33)
                    n930 = call "Set pump parameters.vi"("Pump write delay (ms)"=w1486, "Volume (uL)"="Ch 3 Inject Volume (uL)", "Rate (uL/h)"="Ch 3 Inject Rate (ul/h)", "Units"=4.0, "Pump #"=3.0, "Pump Parameters In"=w1492, "VISA resource name"=w1491) -> ("Pump Parameters Out"=w1484:T33)  [unwired: 3 in]
                    n931 = Bundle By Name(cluster=w1485, "Pump 3"=w1484) -> (w1483:T6)
                    n932 = local write "All Pump Parameters"(w1483) -> ()
                  }
                  frame #1 {
                    n933 = Wait (ms)(milliseconds to wait=w1493) -> ()  [unwired: 1 out]
                  }
                  frame #2 {
                    n934 = call "Write to pump.vi"("string"="start", "VISA resource name"=w1494) -> ()  [unwired: 1 out]
                  }
                  frame #3 {
                    n935 = Wait (ms)(milliseconds to wait=u32 500) -> ()  [unwired: 1 out]
                  }
                  frame #4 {
                    n936 = call "Write to pump.vi"("string"="start", "VISA resource name"=w1498) -> ()  [unwired: 1 out]
                  }
                }
              }
            }
          }
          frame Enabled {
            n937 = call "hamilton_controller.vi"("Open?"=w1500, "valve"=enum16{"A", "B", "C", "D", "ALL"}."A", "action"=T21."MOVE VALVE") -> ()  [unwired: 8 in, 1 out]
          }
        }
      }
      event "Inject Valve B": Value Change {
        n938 = event-data() -> ()  [unwired: 7 out]
        n939 = disable-structure shown="Enabled" {
          disable-tunnel: "Inject Valve B" -> [w1504 w1524]
          frame Disabled {
            n940 = local read "Pump write delay (ms)"() -> (w1506:dbl)
            n941 = flat-sequence {
              tunnel: w1505 -> [w1519]
              tunnel: w1506 -> [w1515]
              tunnel: w1504 -> [_]
              tunnel: w1506 -> [w1521]
              tunnel: w1505 -> [w1522]
              frame #0 {
                n942 = local read "All Pump Parameters"() -> (w1514:T6)
                n943 = Multiply(x=60.0, y="Flush Center Ch Rate (ul/m)") -> (x*y=w1511:dbl)
                n944 = Unbundle By Name(w1514) -> ("Pump 2"=w1520:T33)
                n945 = call "Set pump parameters.vi"("Pump write delay (ms)"=w1515, "Volume (uL)"="Flush Center Ch Volume (uL)", "Rate (uL/h)"=w1511, "Units"=3.0, "Pump #"=2.0, "Pump Parameters In"=w1520, "VISA resource name"=w1519) -> ("Pump Parameters Out"=w1513:T33)  [unwired: 3 in]
                n946 = Bundle By Name(cluster=w1514, "Pump 2"=w1513) -> (w1512:T6)
                n947 = local write "All Pump Parameters"(w1512) -> ()
                n948 = Add(x="Flush Center Ch Volume (uL)", y="Total Volume\nFlushed (uL)") -> (x+y=w1508:dbl)
                n949 = local write "Total Volume\nFlushed (uL)"(w1508) -> ()
              }
              frame #1 {
                n950 = Wait (ms)(milliseconds to wait=w1521) -> ()  [unwired: 1 out]
              }
              frame #2 {
                n951 = call "Write to pump.vi"("string"="start", "VISA resource name"=w1522) -> ()  [unwired: 1 out]
              }
            }
            n952 = local read "Chemyx Syringe Pump Serial Port"() -> (w1505:refnum<visa-resource-name>)
          }
          frame Enabled {
            n953 = call "hamilton_controller.vi"("Open?"=w1524, "valve"=enum16{"A", "B", "C", "D", "ALL"}."B", "action"=T21."MOVE VALVE") -> ()  [unwired: 8 in, 1 out]
          }
        }
      }
      event "Inject Bottom": Value Change {
